vi "Select Target and Engine Dialog.vi"() -> (2 "cancelled?":bool, 3 "engines cluster":T1)   [LabVIEW 2013]
uses:
  <vilib>/NI/Configuration Framework/tree serializer/flat hierarchy.ctl
  <vilib>/NI/Configuration Framework/tree serializer/full hierarchy.ctl
  <vilib>/NI/Configuration Framework/tree serializer/hierarchy element.ctl
  <vilib>/NI/Configuration Framework/tree serializer/instance data.ctl
  <vilib>/NI/Tag Bus Data Framework/Framework Configuration Classes/platypus configuration/engines cluster.ctl
  <vilib>/NI/Module Execution Interface/Engine Configuration/engine configuration.lvclass
  <vilib>/NI/Tag Bus Module Framework/module configuration/TBM module configuration.lvclass
  <vilib>/NI/Configuration Framework/serializable configuration/get alias.vi
  <vilib>/NI/Configuration Framework/tree serializer/NISE_CEF_TreeSerializer.lvlib
  <vilib>/NI/Tag Bus Data Framework/Framework Configuration Classes/flattened data interface/PL_Serialization Interface.lvlib
  <vilib>/NI/Tag Bus Data Framework/Framework Configuration Classes/platypus configuration/PLConfigurationSerializer.lvlib
panel:
  out "data":T2
  in  "Cancel Button":bool
  in  "OK Button":bool
  in  "Engine Selection":string(combo)
  in  "Configuration File Path":path
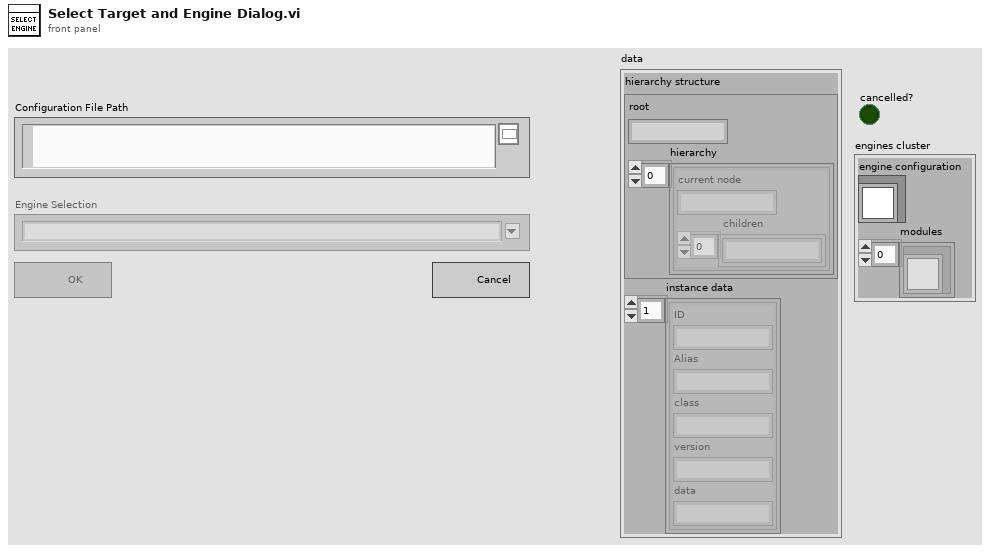
[diagram p1: front panel]
types:
  T1 = typedef "PLConfigurationSerializer.lvlib/engines cluster.ctl" = cluster{"engine configuration":refnum<class "engine configuration.lvclass">, "modules":refnum<class "TBM module configuration.lvclass">[]}
  T2 = typedef "NISE_CEF_TreeSerializer.lvlib/flat hierarchy.ctl" = cluster{"hierarchy structure":T3, "instance data":T5[]}
  T3 = typedef "NISE_CEF_TreeSerializer.lvlib/full hierarchy.ctl" = cluster{"root":string, "hierarchy":T4[]}
  T4 = typedef "NISE_CEF_TreeSerializer.lvlib/hierarchy element.ctl" = cluster{"current node":string, "children":string[]}
  T5 = typedef "NISE_CEF_TreeSerializer.lvlib/instance data.ctl" = cluster{"ID":string, "Alias":string, "class":string, "version":string, "data":string}
  T6 = enum8{"Enabled", "Disabled", "Disabled and Grayed Out"}
  T7 = typedef "NISE_CEF_TreeSerializer.lvlib/base file format.ctl" = cluster{"version":string, "data":string}
  T8 = typedef "PLConfigurationSerializer.lvlib/targets cluster.ctl" = cluster{"Target Configuration":refnum<class "PL_Target Configuration.lvclass">, "engines":T1[]}
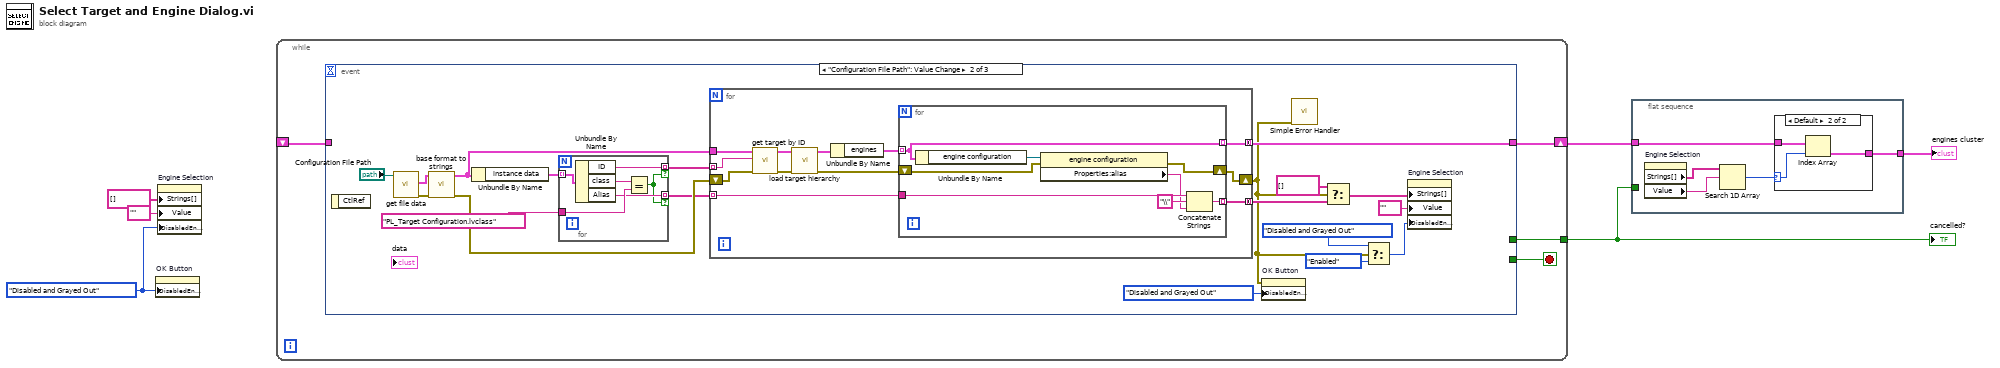
[diagram p0: block diagram]
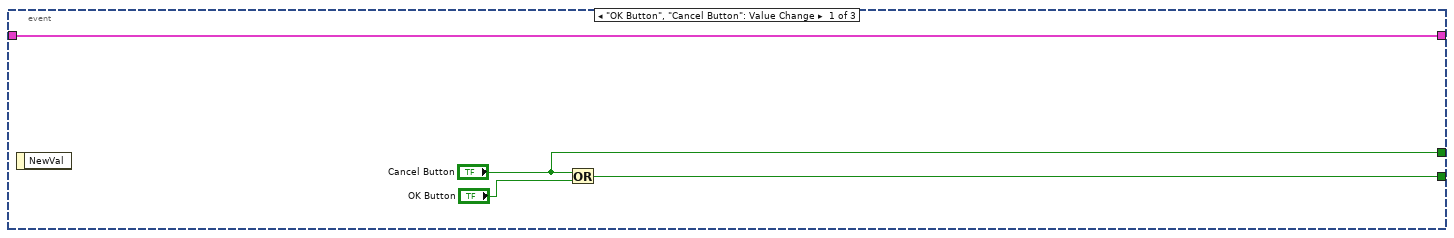
[diagram p3: hidden frame]
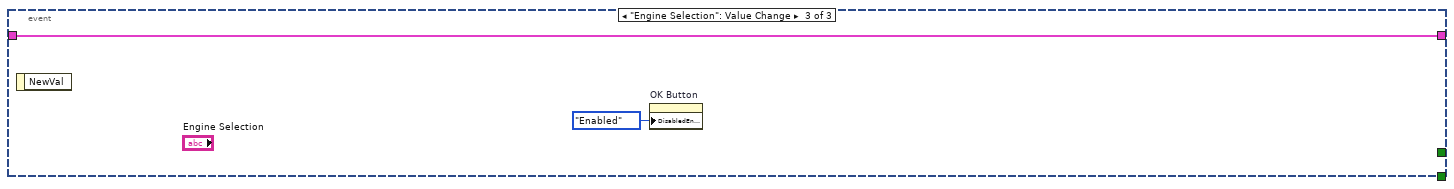
[diagram p4: hidden frame]
diagram:
  w1 = T6."Disabled and Grayed Out" ("Disabled")
  n1 = property on="OK Button" class="Bool"("DisabledEnum"=w1) -> ()  [unwired: 2 in, 2 out]
  n2 = property on="Engine Selection" class="CmbBox"("Strings[]"=string[] [] ("Strings []"), "Value"="" ("Engine Selection"), "DisabledEnum"=w1) -> ()  [unwired: 2 in, 2 out]
  n3 = while {
    tunnel: [w9] -> w3
    shift-right: [w8] -> w5
    shift-left: _ -> [w7]
    stop <- w10 stop-if-true
    n4 = event shown="[1] \"Configuration File Path\": Value Change" {
      selector: _ -> [_ _ _]
      dyn-events: _ -> [_ _ _]
      timeout: _ -> [_ _ _]
      tunnel: [w14 _ _] -> w10
      tunnel: ["Cancel Button" _ _] -> w9
      tunnel: [w11 w24 w60] -> w8
      tunnel: w7 -> [w11 _ w60]
      event "OK Button", "Cancel Button": Value Change {
        n5 = event-data() -> ()  [unwired: 1 in, 1 out]
        n6 = Or(x="Cancel Button", y="OK Button") -> (x .or. y?=w14:bool)
      }
      event "Configuration File Path": Value Change {
        n7 = event-data() -> ()  [unwired: 1 in, 1 out]
        n8 = call <vilib>:"get file data.vi"("Path"="Configuration File Path") -> ("error out"=w32:errorcluster, "format"=w33:T7)  [unwired: 9 in]
        n9 = call <vilib>:"base format to strings.vi"("error in"=w32, "format"=w33) -> ("error out"=w26:errorcluster, "data"=w28:T2)  [unwired: 8 in]
        n10 = Unbundle By Name(w28) -> ("instance data"=w30:T5[])
        n11 = for {
          tunnel: w30 -> [w59] mode=indexing
          tunnel: "PL_Target Configuration.lvclass" -> [w57]
          tunnel: [w56] -> w27 mode=indexing if=w54
          tunnel: [w55] -> w25 mode=indexing if=w54
          n12 = Unbundle By Name(w59) -> ("ID"=w56:string, "class"=w58:string, "Alias"=w55:string)
          n13 = Equal?(x=w58, y=w57) -> (x = y?=w54:bool)
        }
        n14 = for {
          tunnel: w28 -> [w45]
          tunnel: w27 -> [w44] mode=indexing
          shift-right: [w34] -> w16
          shift-left: w26 -> [w41]
          tunnel: w25 -> [w37] mode=indexing
          tunnel: [w38] -> w24 mode=concatenating
          tunnel: [w36] -> w23 mode=concatenating
          n15 = call <vilib>:"get target by ID.vi"("error in"=w41, "UID"=w44, "full system"=w45) -> ("error out"=w42:errorcluster, "target hierarchy"=w43:T2)  [unwired: 7 in]
          n16 = call <vilib>:"load target hierarchy.vi"("error in"=w42, "target hierarchy"=w43) -> ("error out"=w35:errorcluster, "targets cluster out"=w40:T8)  [unwired: 8 in]
          n17 = Unbundle By Name(w40) -> ("engines"=w39:T1[])
          n18 = for {
            tunnel: w39 -> [w46] mode=indexing
            tunnel: [w46] -> w38 mode=indexing
            tunnel: w37 -> [w52]
            tunnel: [w49] -> w36 mode=indexing
            shift-right: [w47] -> w34
            shift-left: w35 -> [w48]
            n19 = Unbundle By Name(w46) -> ("engine configuration"=w53:refnum<class "engine configuration.lvclass">)
            n20 = property class="engine configuration"(reference=w53, error in=w48) -> (error out=w47:errorcluster, "Properties:alias"=w50:string)  [unwired: 1 out]
            n21 = Concatenate Strings(w52, "\\" ("string"), w50) -> (w49:string)
          }
        }
        n22 = property on="OK Button" class="Bool"(error in=w16, "DisabledEnum"=T6."Disabled and Grayed Out" ("Disabled")) -> ()  [unwired: 1 in, 2 out]
        n23 = call <vilib>:"Simple Error Handler.vi"("error in (no error)"=w16) -> ()  [unwired: 4 in, 5 out]
        n24 = Select(t=string[] [], s=w16, f=w23) -> (s? t:f=w19:string[])
        n25 = Select(t=T6."Disabled and Grayed Out" ("Disabled"), s=w16, f=T6."Enabled" ("Disabled")) -> (s? t:f=w15:T6)
        n26 = property on="Engine Selection" class="CmbBox"("Strings[]"=w19, "Value"="" ("Engine Selection"), "DisabledEnum"=w15) -> ()  [unwired: 2 in, 2 out]
      }
      event "Engine Selection": Value Change {
        n27 = event-data() -> ()  [unwired: 1 in, 1 out]
        n28 = property on="OK Button" class="Bool"("DisabledEnum"=T6."Enabled" ("Disabled")) -> ()  [unwired: 2 in, 2 out]
      }
    }
  }
  "cancelled?" <- w3
  n29 = flat-sequence {
    tunnel: w3 -> [_]
    tunnel: w5 -> [w63]
    tunnel: [w62] -> w4
    frame #0 {
      n30 = property on="Engine Selection" class="CmbBox"() -> ("Strings[]"=w66:string[], "Value"=w65:string)  [unwired: 2 in, 2 out]
      n31 = Search 1D Array(1D array=w66, element=w65) -> (index of element=w64:i32)  [unwired: 1 in]
      n32 = case shown="Default" w64 {
        selector: w64 -> [_ w68]
        tunnel: w63 -> [_ w69]
        tunnel: [_ w67] -> w62
        frame -1 {
        }
        frame Default {
          n33 = Index Array(array=w69, index=w68) -> (element=w67:T1)
        }
      }
    }
  }
  "engines cluster" <- w4
